vi "initializeProgram.vi"(11 "vi folder":path) -> ()   [LabVIEW 2015]
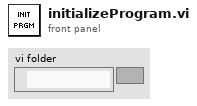
[diagram p1: front panel]
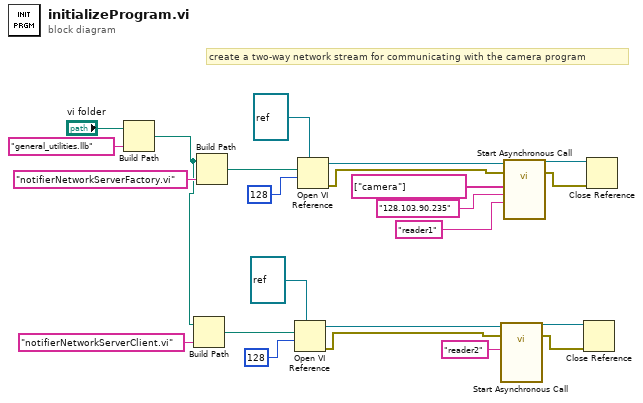
[diagram p0: block diagram]
diagram:
  # "create a two-way network stream for communicating with the camera program"
  n1 = Build Path(base path="vi folder", name or relative path="general_utilities.llb") -> (appended path=w2:path)
  n2 = Build Path(base path=w2, name or relative path="notifierNetworkServerClient.vi") -> (appended path=w8:path)
  n3 = Build Path(base path=w2, name or relative path="notifierNetworkServerFactory.vi") -> (appended path=w19:path)
  n4 = Open VI Reference(type specifier VI Refnum (for type only)=refnum<vi> refnum, vi path=w8, options=128) -> (vi reference=w9:refnum<vi>, error out=w5:errorcluster)  [unwired: 3 in]
  n5 = Open VI Reference(type specifier VI Refnum (for type only)=refnum<vi> refnum, vi path=w19, options=128) -> (vi reference=w20:refnum<vi>, error out=w13:errorcluster)  [unwired: 3 in]
  n6 = call-by-ref "Start Asynchronous Call"(reference=w9, error in=w5, "reader name"="reader2") -> (reference out=w7:refnum<vi>, error out=w6:errorcluster)  [unwired: 11 in]
  n7 = call-by-ref "Start Asynchronous Call"(reference=w20, error in=w13, "reader name"="reader1", "ip address"="128.103.90.235", "notifier names"=string[] ["camera"]) -> (reference out=w15:refnum<vi>, error out=w14:errorcluster)  [unwired: 9 in]
  n8 = Close Reference(reference=w7, error in (no error)=w6) -> ()  [unwired: 1 out]
  n9 = Close Reference(reference=w15, error in (no error)=w14) -> ()  [unwired: 1 out]
